vi "entropy_cal_optic_sub.vi"(1 "T_1D":i32[](array[numeric]), 2 "Y_1D":ext[](array[numeric])=[0.0, 0.0, 0.0, 0.0, 0.0, 0.0, 0.0, 0.0, 0.0, 0.0, 0.0, 0.0, 0.0, 0.0, 0.0, 0.0, 0.0, 0.0, 0.0, 0.0, 0.0, 0.0, 0.0, 0.0, 0.0, 0.0, 0.0]) -> (0 "Entropy":ext)   [LabVIEW 2021]
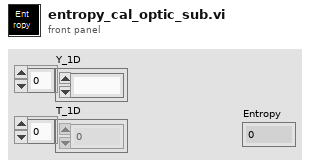
[diagram p1: front panel]
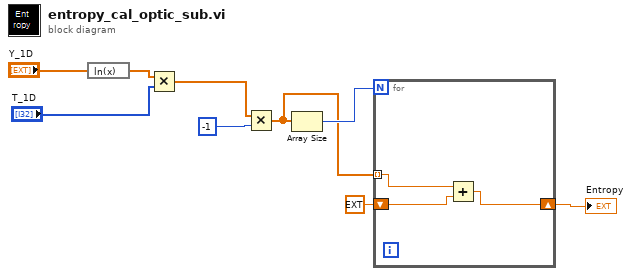
[diagram p0: block diagram]
diagram:
  n1 = expression code="ln(x)"("Y_1D") -> (w8:ext[])
  n2 = Multiply(x=w8, y="T_1D") -> (x*y=w6:ext[])
  n3 = Multiply(x=w6, y=-1) -> (x*y=w3:ext[])
  n4 = Array Size(array=w3) -> (size(s)=w4:i32)
  n5 = for {
    N: w4 -> [_]
    tunnel: w3 -> [w12] mode=indexing
    shift-right: [w11] -> w1
    shift-left: ext 0.0 -> [w10]
    n6 = Add(x=w12, y=w10) -> (x+y=w11:ext)
  }
  "Entropy" <- w1
